vi "WritePanelData.vi"(8 "error in (no error)":errorcluster, 10 "Panel Data Array":T1[](array[typedef]), 11 "MAUI in":refnum<class "SMO.UI.MAUI.lvclass">) -> (0 "error out":errorcluster, 3 "MAUI out":refnum<class "SMO.UI.MAUI.lvclass">)   [LabVIEW 2019, in "SMO.UI.MAUI.lvclass"]
uses:
  SMO.UI.MAUI.lvclass
  Typedefs/PanelData.ctl
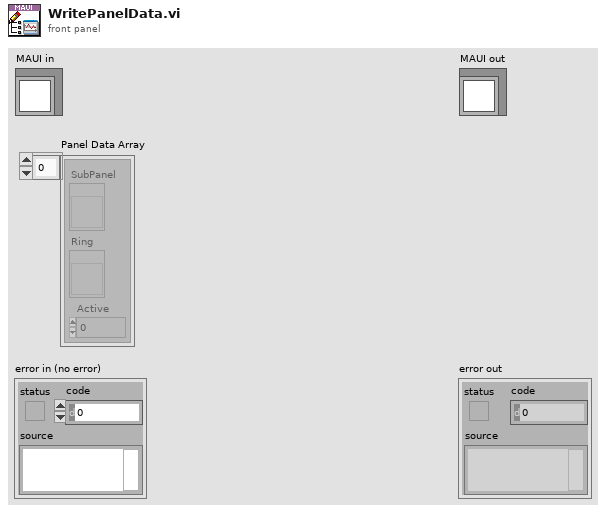
[diagram p1: front panel]
types:
  T1 = typedef "SMO.UI.MAUI.lvclass/PanelData.ctl" = cluster{"SubPanel":refnum<vi>, "Ring":refnum<vi>, "Active":i32}
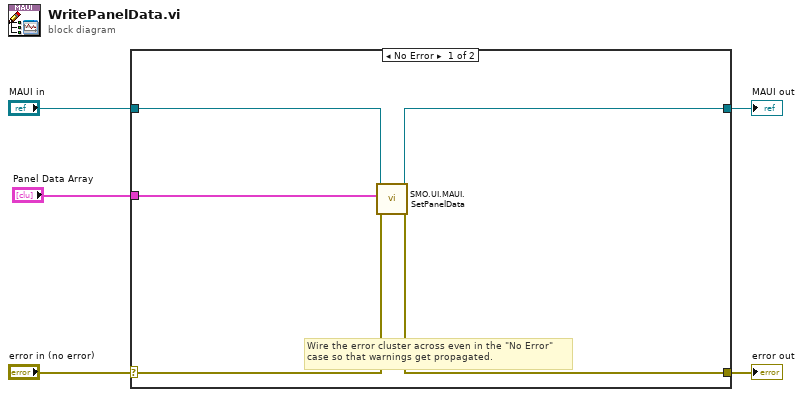
[diagram p0: block diagram]
diagram:
  n1 = case shown="No Error" "error in (no error)" {
    selector: "error in (no error)" -> [w7 w12]
    tunnel: [w6 w12] -> w4
    tunnel: [w8 w11] -> w2
    tunnel: "MAUI in" -> [w9 w11]
    tunnel: "Panel Data Array" -> [w10 _]
    frame No Error {
      # "Wire the error cluster across even in the \"No Error\"\ncase so that warnings get propagated."
      n2 = call "SMO.UI.MAUI.SetPanelData.vi"("error in (no error)"=w7, "SetPanelData"=w10, "MAUI"=w9) -> ("error out"=w6:errorcluster, "MAUI out"=w8:refnum<class "SMO.UI.MAUI.lvclass">)  [unwired: 7 in]
    }
    frame Error {
    }
  }
  "error out" <- w4
  "MAUI out" <- w2
